vi "get Optimised Texture Pointer.vi"(11 "Texture in":refnum<class "Texture.lvclass">) -> (3 "Optimised Texture Pointer":u32 format="%.0x")   [LabVIEW 2021, in "Texture.lvclass"]
uses:
  Texture.lvclass
  Texture.lvclass/Texture.ctl
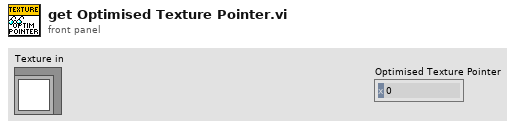
[diagram p1: front panel]
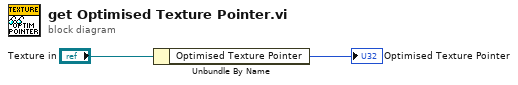
[diagram p0: block diagram]
diagram:
  n1 = Unbundle By Name("Texture in") -> ("Optimised Texture Pointer"=→"Optimised Texture Pointer":u32)
